vi "for loop.vi"() -> ()   [LabVIEW 2020]
panel:
  out "Array 6":dbl[](array[numeric])=[0.0, 1.0, 2.0, 3.0]
  in  "Array 5":dbl[](array[numeric])
  out "Array 4":dbl[](array[numeric])
  out "Numeric 6":i32
  out "Numeric 5":dbl
  out "Numeric 4":i32
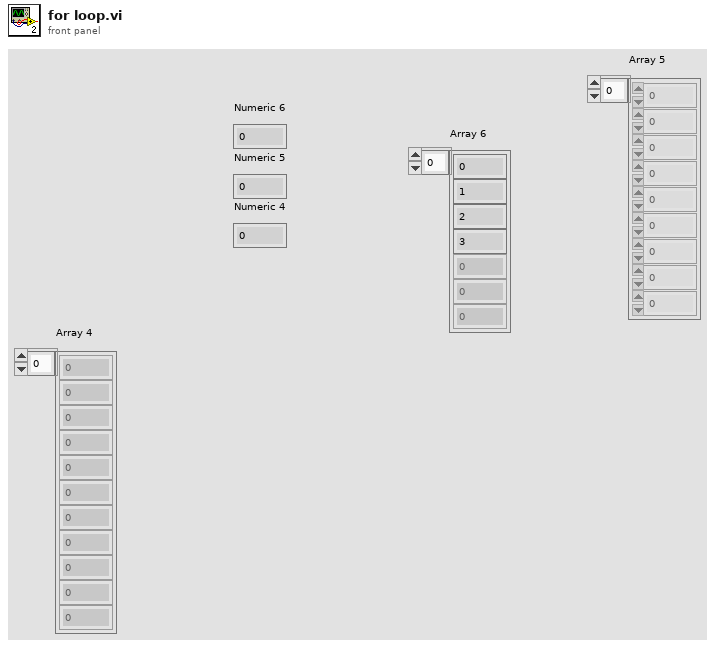
[diagram p1: front panel]
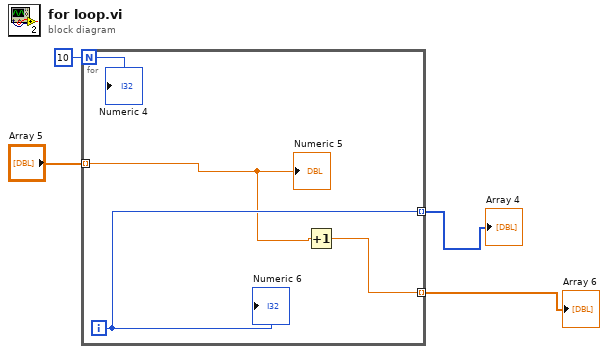
[diagram p0: block diagram]
diagram:
  n1 = for {
    N: 10 -> [w7]
    tunnel: [w8] -> w3 mode=indexing
    tunnel: "Array 5" -> [w6] mode=indexing
    tunnel: [w5] -> w1 mode=indexing
    i -> [w8]
    n2 = Increment(x=w6) -> (x+1=w5:dbl)
    "Numeric 6" <- w8
    "Numeric 5" <- w6
    "Numeric 4" <- w7
  }
  "Array 4" <- w3
  "Array 6" <- w1
